vi "Play With Picture.vi"() -> ()   [LabVIEW 2014]
panel:
  out "2D Picture":picture
  out "bmp image vector":dbl[](array[numeric])
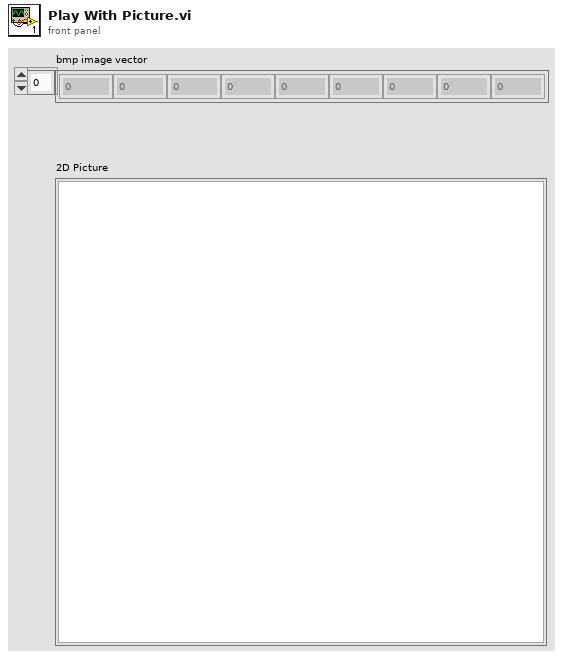
[diagram p1: front panel]
types:
  T1 = typedef "imagedata.ctl" = cluster{"image type":i32, "image depth":i32, "image":u8[], "mask":u8[], "colors":u32[], "Rectangle":cluster{"left":i16, "top":i16, "right":i16, "bottom":i16}}
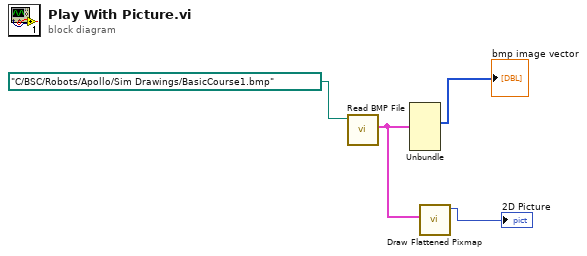
[diagram p0: block diagram]
diagram:
  n1 = call <vilib>:"Read BMP File.vi"("path to BMP file"=path "C:/BSC/Robots/Apollo/Sim Drawings/BasicCourse1.bmp") -> ("image data"=w2:T1)  [unwired: 8 in, 2 out]
  n2 = Unbundle(w2) -> ("image"=→"bmp image vector":u8[])  [unwired: 5 out]
  n3 = call <vilib>:"Draw Flattened Pixmap.vi"("image data"=w2) -> ("new picture"=→"2D Picture":picture)  [unwired: 8 in]
